vi "SubVI - Receive File.vi"(11 "file path (use dialog)":path) -> (0 "error out":errorcluster)   [LabVIEW 2017]
uses:
  Global/Test_Selection.vi
panel:
  out "Progress ( % )":u8
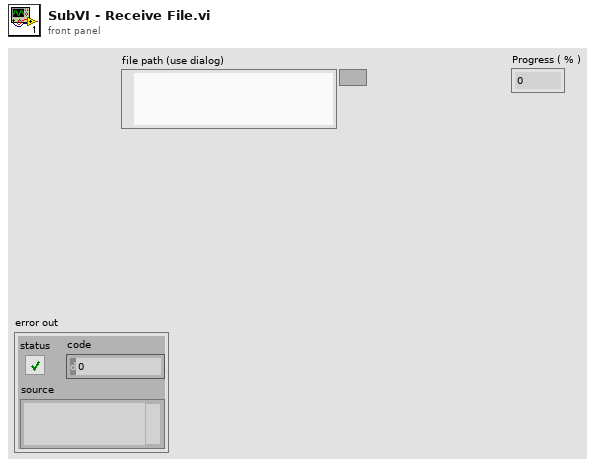
[diagram p1: front panel]
types:
  T1 = enum16{"open", "replace", "create", "open or create", "replace or create", "replace or create with confirmation"}
  T2 = enum16{"big-endian, network order", "native, host order", "little-endian"}
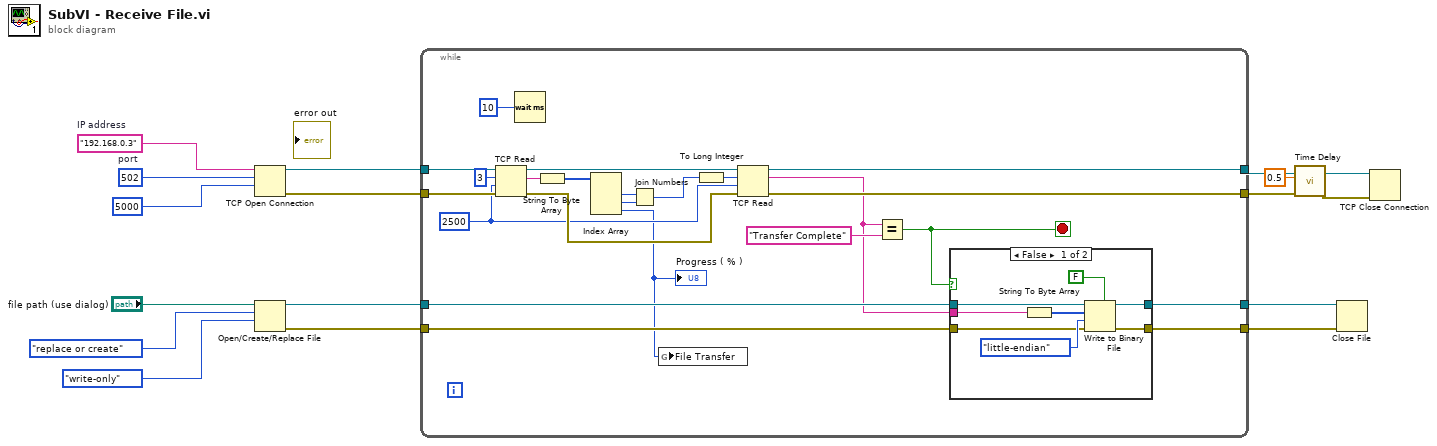
[diagram p0: block diagram]
diagram:
  w15 = u16 502  # port
  w16 = "192.168.0.3"  # IP address
  n1 = TCP Open Connection(address=w16, remote port or service name=w15, timeout ms (60000)=5000 ("timeout ms (wait forever: -1)")) -> (connection ID=w13:refnum<k5>, error out=w12:errorcluster)  [unwired: 2 in]
  n2 = Open/Create/Replace File(file path (use dialog)="file path (use dialog)", operation (0:open)=T1."replace or create", access (0:read/write)=enum16{"read/write", "read-only", "write-only"}."write-only") -> (refnum out=w5:refnum<file>, error out=w6:errorcluster)  [unwired: 3 in, 1 out]
  n3 = while {
    tunnel: w13 -> [w39]
    tunnel: w12 -> [w38]
    tunnel: [w29] -> w11
    tunnel: [w28] -> w10
    tunnel: w6 -> [w25]
    tunnel: w5 -> [w24]
    tunnel: [w23] -> w4
    tunnel: [w22] -> w3
    stop <- w20 stop-if-true
    w18 = 2500 ("timeout ms (25000)")
    n4 = TCP Read(connection ID=w39, bytes to read=3, error in (no error)=w38, 9:w18) -> (connection ID out=w32:refnum<k5>, data out=w36:string, error out=w31:errorcluster)  [unwired: 1 in]
    n5 = Wait (ms)(milliseconds to wait=u32 10) -> ()  [unwired: 1 out]
    n6 = String To Byte Array(string=w36) -> (unsigned byte array=w35:u8[])
    n7 = Index Array(array=w35) -> (element #1=w34:u8, element #2=w33:u8, element #3=w17:u8)  [unwired: 3 in]
    "Progress ( % )" <- w17
    n8 = Join Numbers(hi=w34, lo=w33) -> ((hi.lo)=w19:u16)
    n9 = global write "Test_Selection.vi" "File Transfer"(w17) -> ()
    n10 = To Long Integer(number=w19) -> (32bit integer=w30:i32)
    n11 = TCP Read(connection ID=w32, bytes to read=w30, error in (no error)=w31, 9:w18) -> (connection ID out=w29:refnum<k5>, data out=w21:string, error out=w28:errorcluster)  [unwired: 1 in]
    n12 = Equal?(x=w21, y="Transfer Complete" ("data in")) -> (x = y?=w20:bool)
    n13 = case shown="False" w20 {
      tunnel: w25 -> [w45 w48]
      tunnel: w24 -> [w44 w49]
      tunnel: [w43 w49] -> w23
      tunnel: [w42 w48] -> w22
      tunnel: w21 -> [w41 _]
      frame False {
        n14 = String To Byte Array(string=w41) -> (unsigned byte array=w40:u8[])
        n15 = Write to Binary File(file (use dialog)=w44, data=w40, error in=w45, 5:FALSE ("prepend array or string size? (T)"), 9:T2."little-endian" ("byte order (0:big-endian, network order)")) -> (refnum out=w43:refnum<file>, error out=w42:errorcluster)  [unwired: 1 in, 1 out]
      }
      frame True {
      }
    }
  }
  n16 = call "Time Delay"("error in (no error)"=w10, "Delay Time (s)"=0.5) -> ("error out"=w2:errorcluster)  [unwired: 9 in]
  n17 = Close File(refnum=w4, error in=w3) -> ()  [unwired: 2 out]
  n18 = TCP Close Connection(connection ID=w11, error in (no error)=w2) -> ()  [unwired: 1 in, 2 out]
